vi "adam-digital-outputs.vi"(0 "VISA Refnum in":refnum<visa-resource-name>, 1 "Chassis Settings":T2, 5 "Current DO State":T1, 7 "DO Control":T1, 9 "chassis-slot":i32, 11 "error in (no error)":errorcluster, 12 "cmd-in":string, 13 "ack char":string) -> (4 "VISA Refnum out":refnum<visa-resource-name>, 6 "New DO State":T1, 8 "cmd-out":string, 10 "acknowledge char":string, 14 "cmd aknowledged":bool, 15 "error out":errorcluster)   [LabVIEW 2020]
uses:
  controls/digital-output-cluster.ctl
  controls/adam-5000-serial-settings.ctl
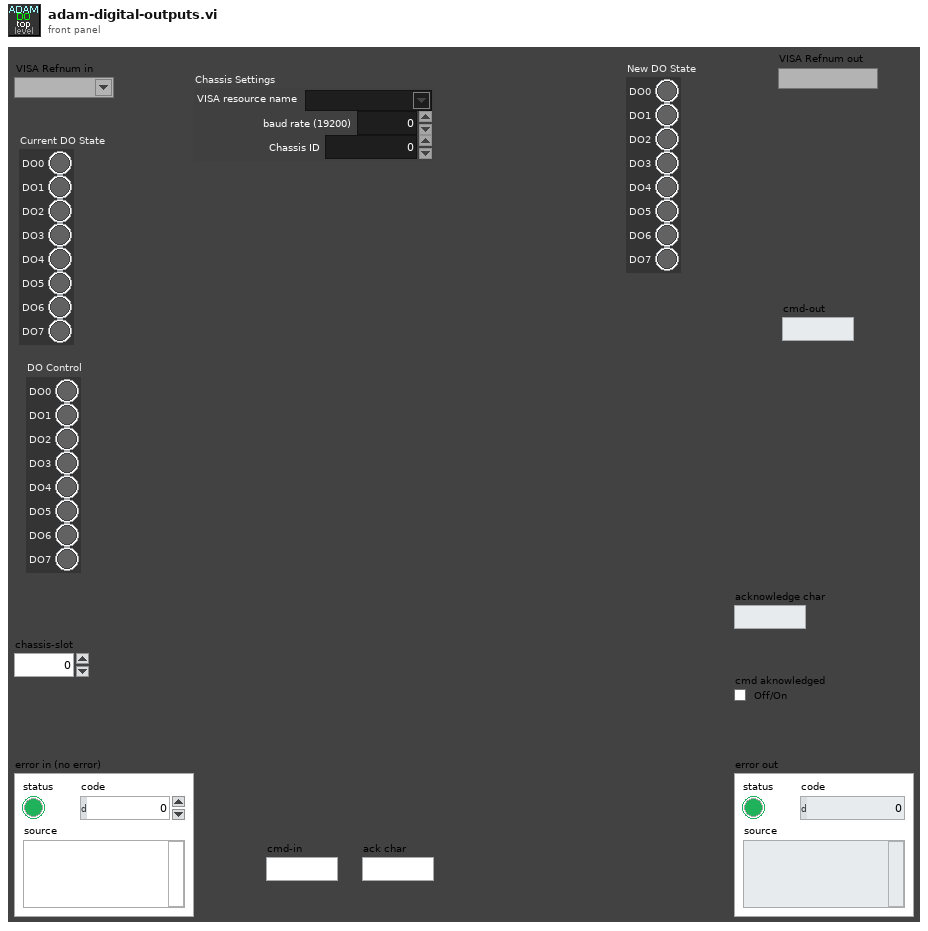
[diagram p1: front panel]
types:
  T1 = typedef "digital-output-cluster.ctl" = cluster{"DO0":bool, "DO1":bool, "DO2":bool, "DO3":bool, "DO4":bool, "DO5":bool, "DO6":bool, "DO7":bool}
  T2 = typedef "adam-5000-serial-settings.ctl" = cluster{"VISA resource name":refnum<visa-resource-name>, "baud rate (19200)":u32, "Chassis ID":u8}
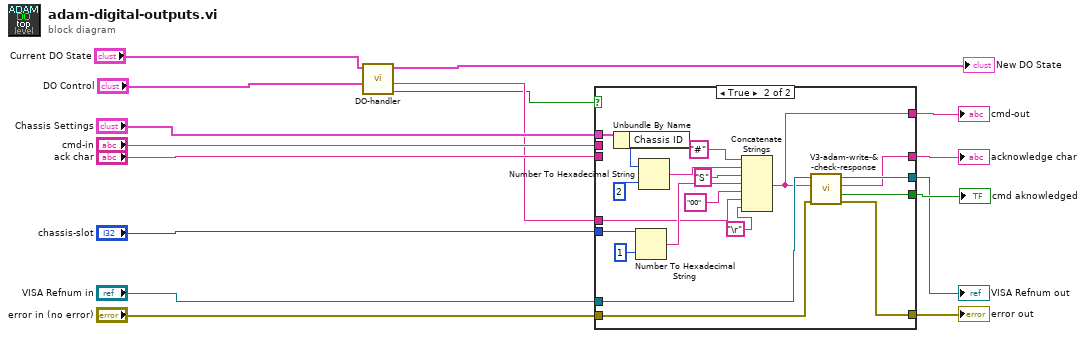
[diagram p0: block diagram]
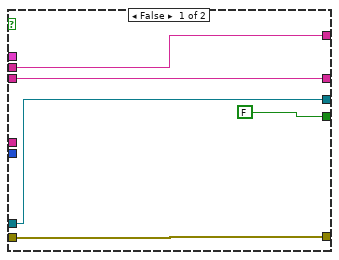
[diagram p2: hidden frame]
diagram:
  n1 = call "DO-handler.vi"("Output Control"="DO Control", "Current Output State"="Current DO State") -> ("output state changed"=w4:bool, "hex integer string"=w5:string, "DO Output"=→"New DO State":T1)  [unwired: 5 in, 2 out]
  n2 = case shown="True" w4 {
    tunnel: w5 -> [_ w31]
    tunnel: "Chassis Settings" -> [_ w40]
    tunnel: "chassis-slot" -> [_ w35]
    tunnel: "VISA Refnum in" -> [w21 w29]
    tunnel: "error in (no error)" -> [w19 w28]
    tunnel: [w19 w27] -> w10
    tunnel: [w21 w26] -> w11
    tunnel: [FALSE ("cmd aknowledged") w25] -> w14
    tunnel: [w18 w24] -> w12
    tunnel: "ack char" -> [w18 _]
    tunnel: [w17 w23] -> w15
    tunnel: "cmd-in" -> [w17 _]
    frame False {
    }
    frame True {
      n3 = Unbundle By Name(w40) -> ("Chassis ID"=w39:u8)
      n4 = Number To Hexadecimal String(1:i16 1 ("width (-)"), 2:w35) -> (0:w33:string)
      n5 = Number To Hexadecimal String(1:i16 2 ("width (-)"), 2:w39) -> (0:w37:string)
      n6 = Concatenate Strings("#" ("string"), w37, "S" ("string"), w33, "00" ("string"), w31, "\r") -> (w23:string)
      n7 = call "V3-adam-write-&-check-response.vi"("error in (no error)"=w28, "write buffer"=w23, "VISA resource name"=w29) -> ("error out"=w27:errorcluster, "cmd aknowledged"=w25:bool, "acknowledge char"=w24:string, "VISA resource name out"=w26:refnum<visa-resource-name>)  [unwired: 4 in, 1 out]
    }
  }
  "cmd-out" <- w15
  "cmd aknowledged" <- w14
  "acknowledge char" <- w12
  "VISA Refnum out" <- w11
  "error out" <- w10
